vi "saveBackground.vi"(11 "im proc controls":T1={"Color Plane"=2, "downsampling"=24, "Filter"=enum."AutoM", "Number of Erosions"=2, "Focus threshold"=20.0, "Focus std threshold"=0.0, "background\nsubtraction"=FALSE, "Threshold"=0} {"Threshold" scale=0.0..255.0; "Color Plane" items=["Red", "Green", "Blue", "Hue", "Saturation", "Luminance", "Value", "Intensity"]}) -> ()   [LabVIEW 2012]
uses:
  GlobalBaslerCamera.vi
  Cpp Libraries/CatWalkLabviewDLL/labview code/OpenCvGlobals.vi
  <resource>/objmgr/imaqdx.rc
  <vilib>/vision/driver/NI_Vision_Acquisition_Software.lvlib
  <vilib>/vision/NI_Vision_Development_Module.lvlib
panel:
  in  "Number of frames":i64=16
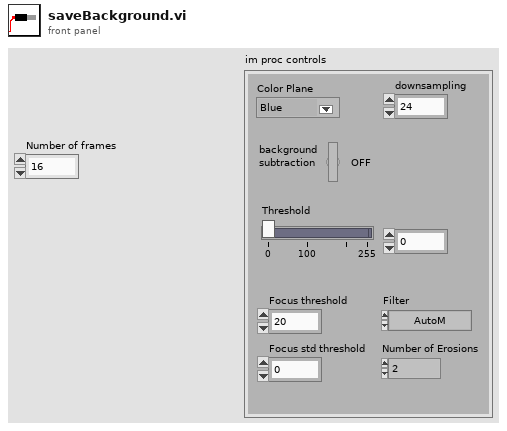
[diagram p1: front panel]
types:
  T1 = cluster{"Color Plane":i32, "downsampling":i32, "Filter":enum32{"AutoM", "Close", "Dilate", "Erode", "Gradient", "Gradient out", "Gradient in", "Hit miss", "Open", "PClose", "POpen", "Thick", "Thin"}, "Number of Erosions":i32, "Focus threshold":sgl, "Focus std threshold":sgl, "background\nsubtraction":bool, "Threshold":u8}
  T2 = typedef "IMAQ Image.ctl" = refnum<image>
  T3 = typedef "IMAQdx.ctl" = refnum<k21>
  T4 = typedef "Semaphore RefNum" = refnum<k1>
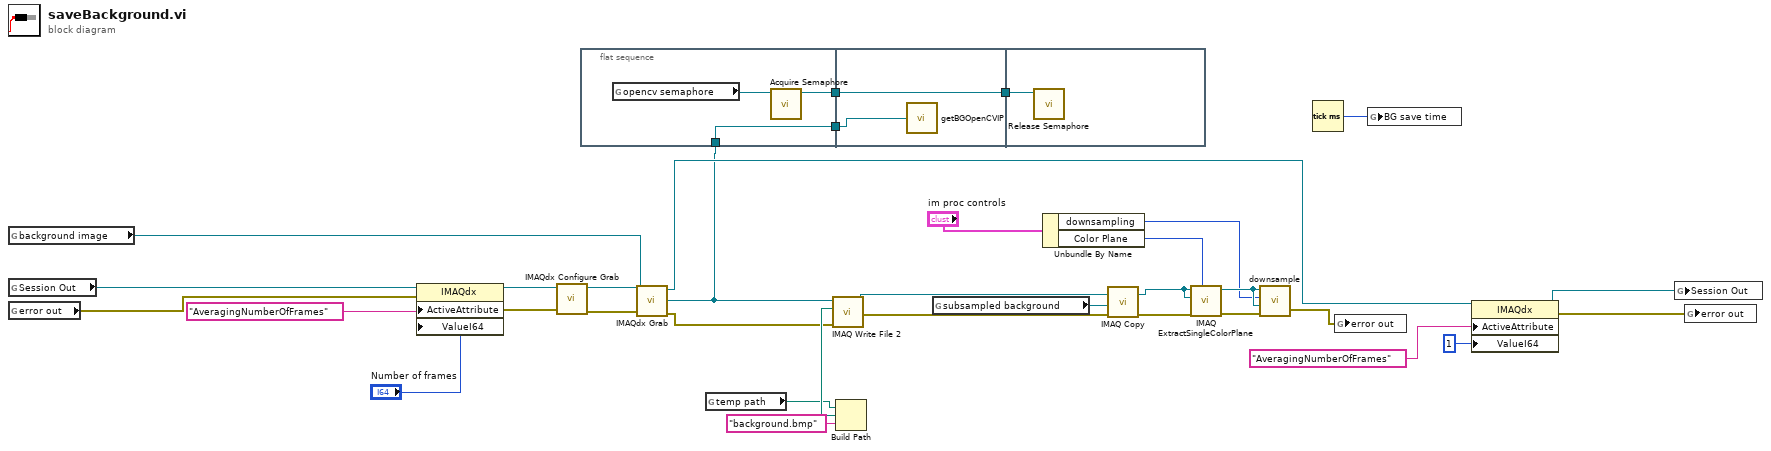
[diagram p0: block diagram]
diagram:
  n1 = global read "GlobalBaslerCamera.vi" "background image"() -> (w17:T2)
  n2 = global read "GlobalBaslerCamera.vi" "Session Out"() -> (w26:T3)
  n3 = global read "GlobalBaslerCamera.vi" "error out"() -> (w25:errorcluster)
  n4 = property class="IMAQdx"(reference=w26, error in=w25, "ActiveAttribute"="AveragingNumberOfFrames", "ValueI64"="Number of frames") -> (reference out=w34:T3, error out=w33:errorcluster)
  n5 = call <vilib>:"IMAQdx Configure Grab.vi"("error in"=w33, "Session In"=w34) -> ("error out"=w29:errorcluster, "Session Out"=w30:T3)  [unwired: 8 out]
  n6 = flat-sequence {
    tunnel: [w36] -> w7
    tunnel: w5 -> [w35]
    tunnel: [w35] -> w4
    tunnel: w7 -> [w39]
    tunnel: [w39] -> w6
    tunnel: w4 -> [w38]
    tunnel: w6 -> [w40]
    frame #0 {
      n7 = global read "OpenCvGlobals.vi" "opencv semaphore"() -> (w37:T4)
      n8 = call <vilib>:"Acquire Semaphore.vi"("semaphore"=w37) -> ("semaphore out"=w36:T4)  [unwired: 4 in, 2 out]
    }
    frame #1 {
      n9 = call "getBGOpenCVIP.vi"("Image"=w38) -> ()  [unwired: 1 out]
    }
    frame #2 {
      n10 = call <vilib>:"Release Semaphore.vi"("semaphore"=w40) -> ()  [unwired: 5 in, 2 out]
    }
  }
  n11 = call <vilib>:"IMAQdx Grab.vi"("error in"=w29, "Image In"=w17, "Session In"=w30) -> ("error out"=w18:errorcluster, "Image Out"=w5:T2, "Session Out"=w24:T3)  [unwired: 5 in, 1 out]
  n12 = global read "GlobalBaslerCamera.vi" "temp path"() -> (w20:path)
  n13 = Build Path(base path=w20, name or relative path="background.bmp") -> (appended path=w21:path)
  n14 = call-poly "IMAQ Write File 2"("error in (no error)"=w18, "File Path"=w21, "Image"=w5) -> ("error out"=w14:errorcluster, "Image Out (duplicate)"=w15:T2)  [unwired: 7 in]
  n15 = global read "GlobalBaslerCamera.vi" "subsampled background"() -> (w16:T2)
  n16 = Unbundle By Name("im proc controls") -> ("downsampling"=w10:i32, "Color Plane"=w9:i32)
  n17 = call "IMAQ Copy"("error in (no error)"=w14, "Image Dst"=w16, "Image Src"=w15) -> ("error out"=w3:errorcluster, "Image Dst Out"=w12:T2)  [unwired: 3 in]
  n18 = call "IMAQ ExtractSingleColorPlane"("Color Plane"=w9, "error in (no error)"=w3, "Image Dst"=w12, "Image Src"=w12) -> ("error out"=w2:errorcluster, "Image Dst Out"=w13:T2)  [unwired: 6 in]
  n19 = call "downsample.vi"("error in"=w2, "img dst"=w13, "downsampling"=w10, "img src"=w13) -> ("error out"=w1:errorcluster)  [unwired: 1 out]
  n20 = Tick Count (ms)() -> (millisecond timer value=w8:u32)
  n21 = global write "GlobalBaslerCamera.vi" "error out"(w1) -> ()
  n22 = global write "GlobalBaslerCamera.vi" "BG save time"(w8) -> ()
  n23 = property class="IMAQdx"(reference=w24, "ActiveAttribute"="AveragingNumberOfFrames", "ValueI64"=i64 1 ("Number of frames 2")) -> (reference out=w23:T3, error out=w22:errorcluster)  [unwired: 1 in]
  n24 = global write "GlobalBaslerCamera.vi" "Session Out"(w23) -> ()
  n25 = global write "GlobalBaslerCamera.vi" "error out"(w22) -> ()
